vi "SwerveDriveTwoDrivers.vi"(0 "Strafe Joystick Axes":cluster{"X":dbl, "Y":dbl}, 1 "Face Joystick Axes":cluster{"X":dbl, "Y":dbl}, 2 "Trigger Axes":cluster{"output":dbl, dbl}, 3 "Face PID Gains":T2 {"derivative time (Td, min)" format="%.3f"; "integral time (Ti, min)" format="%.3f"; "proportional gain (Kc)" format="%.3f"}, 4 "Angle (degrees; 0 = right)":dbl, 5 "error in (no error)":errorcluster, 6 "Strafe Multiplier":dbl, 8 "Rotation Multiplier":dbl, 9 "ArmCRotates?":bool, 10 "Max Wheel Speed":dbl) -> (19 "error out":errorcluster)   [LabVIEW 2014]
uses:
  <vilib>/addons/control/pid/pid.llb/PID Control Input Filter (DBL).vi
  <vilib>/addons/control/pid/pid.llb/PID (DBL).vi
  <vilib>/addons/control/pid/NI_PID_pid.lvlib
panel:
  out "diff.":dbl
  out "Waveform Chart":T1(graph)
  out "Robot Heading":dbl(knob) scale=3.1416..-3.1416
  out "Joystick Angle":dbl(knob) scale=3.1416..-3.1416
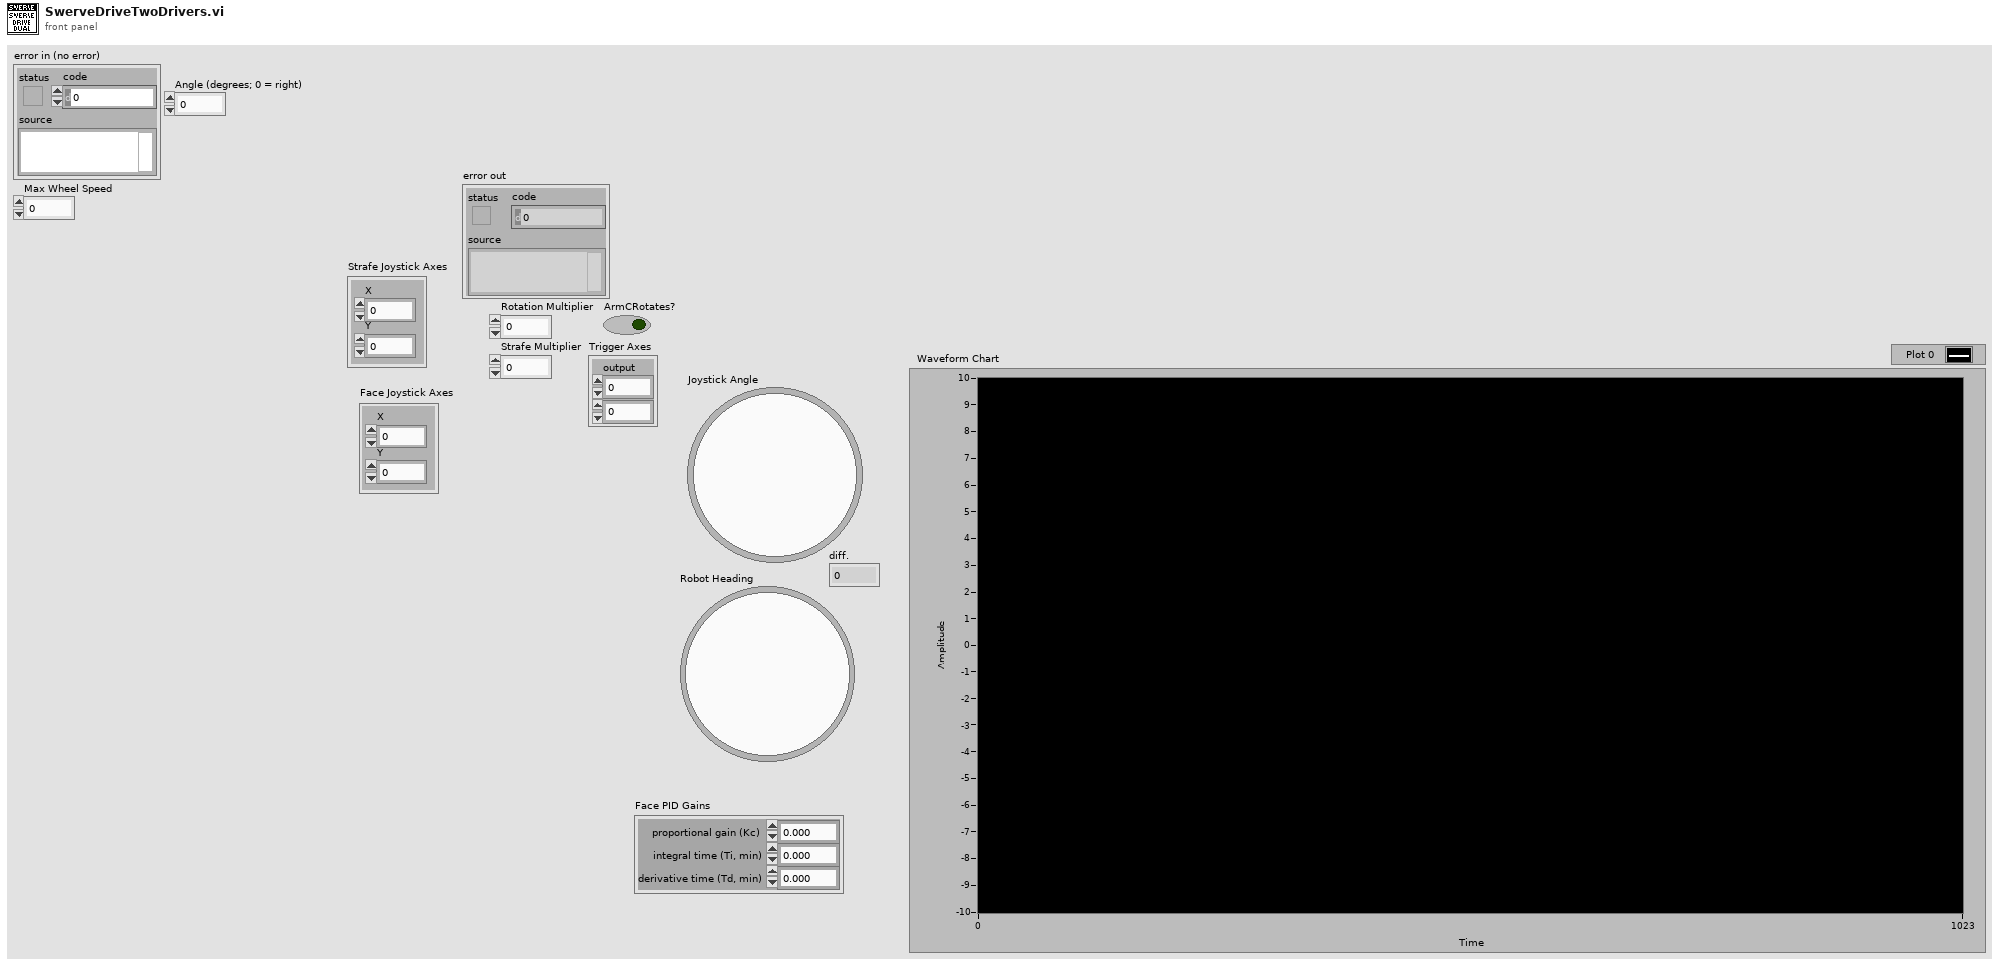
[diagram p1: front panel]
types:
  T1 = cluster{"output":dbl, "output":dbl, "millisecond timer value":u32}
  T2 = cluster{"proportional gain (Kc)":dbl, "integral time (Ti, min)":dbl, "derivative time (Td, min)":dbl}
  T3 = cluster{"output angle":dbl, "output":dbl, "millisecond timer value":u32}
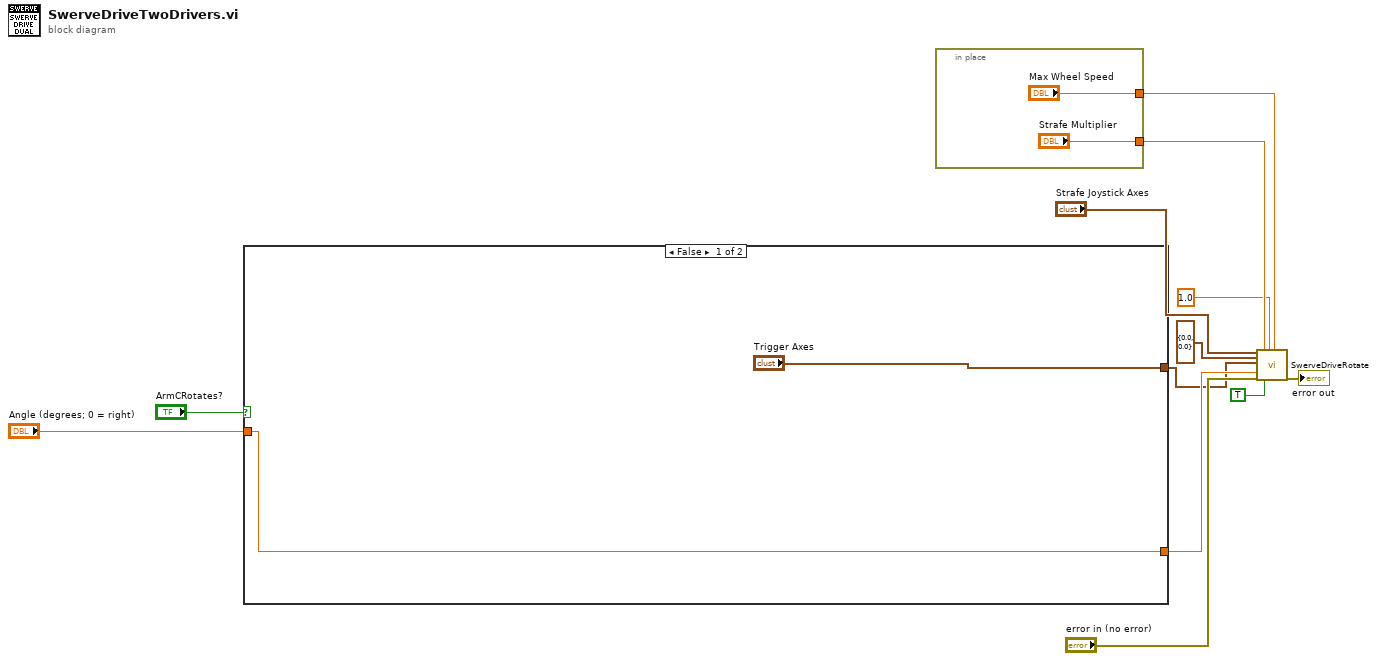
[diagram p0: block diagram]
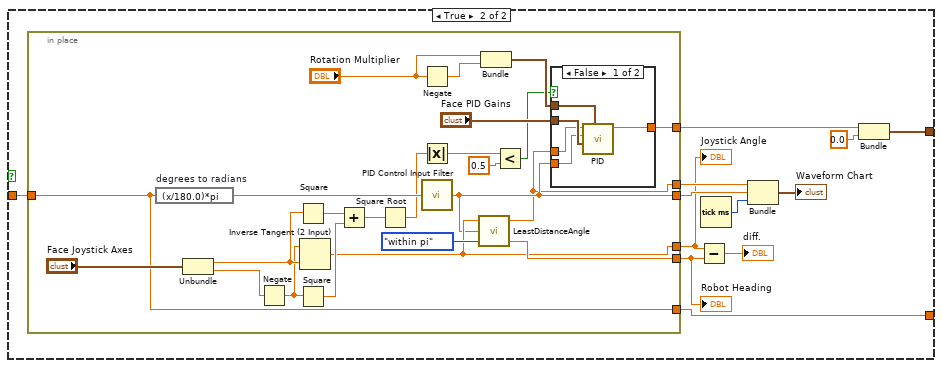
[diagram p2: hidden frame]
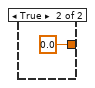
[diagram p3: hidden frame]
diagram:
  n1 = case shown="False" "ArmCRotates?" {
    tunnel: ["Trigger Axes" w24] -> w1
    tunnel: [w14 w23] -> w11
    tunnel: "Angle (degrees; 0 = right)" -> [w14 w15]
    frame False {
    }
    frame True {
      n2 = in-place {
        in-place-border: [w49] -> w25
        in-place-border: [w27] -> w23
        in-place-border: [w31] -> w18
        in-place-border: [w33] -> w17
        in-place-border: [w29] -> w20
        in-place-border: [w28] -> w19
        in-place-border: w15 -> [w27]
        n3 = expression code="(x/180.0)*pi" "degrees to radians"(w27) -> (w46:dbl)
        n4 = Unbundle("Face Joystick Axes") -> ("X"=w41:dbl, "Y"=w40:dbl)
        n5 = Negate(x=w40) -> (-x=w37:dbl)
        n6 = Square(x=w41) -> (x^2=w45:dbl)
        n7 = Square(x=w37) -> (x^2=w44:dbl)
        n8 = Inverse Tangent (2 Input)(1:w41, 2:w37) -> (0:w31:dbl)
        n9 = Add(x=w45, y=w44) -> (x+y=w43:dbl)
        n10 = Square Root(x=w43) -> (sqrt(x)=w42:dbl)
        n11 = Negate(x="Rotation Multiplier") -> (-x=w35:dbl)
        n12 = Absolute Value(x=w42) -> (abs(x)=w38:dbl)
        n13 = call-poly <vilib>:"PID Control Input Filter.vi"("input"=w46) -> ("output"=w29:dbl)  [unwired: 4 in]
        n14 = call "LeastDistanceAngle.vi"("Enum"=enum16{"within pi", "within pi/2"}."within pi", "Current angle"=w29, "target angle (between pi and -pi) 2"=w31) -> ("current angle (between pi and -pi) 2"=w33:dbl, "output angle"=w28:dbl)  [unwired: 1 out]
        n15 = Bundle("Rotation Multiplier"="Rotation Multiplier", w35) -> (w34:cluster{"Rotation Multiplier":dbl, dbl})  [unwired: 1 in]
        n16 = Less?(x=w38, y=0.5) -> (x < y?=w30:bool)
        n17 = case shown="False" w30 {
          tunnel: [w54 0.0 ("output")] -> w49
          tunnel: "Face PID Gains" -> [w53 _]
          tunnel: w34 -> [w52 _]
          tunnel: w29 -> [w51 _]
          tunnel: w28 -> [w50 _]
          frame False {
            n18 = call-poly <vilib>:"PID.vi"("output range"=w52, "PID gains"=w53, "process variable"=w51, "setpoint"=w50) -> ("output"=w54:dbl)  [unwired: 6 in, 1 out]
          }
          frame True {
          }
        }
      }
      "Joystick Angle" <- w18
      "Robot Heading" <- w17
      n19 = Subtract(x=w18, y=w17) -> (x-y=→"diff.":dbl)
      n20 = Tick Count (ms)() -> (millisecond timer value=w22:u32)
      n21 = Bundle("output angle"=w19, "output"=w20, "millisecond timer value"=w22) -> (→"Waveform Chart":T3)  [unwired: 1 in]
      n22 = Bundle("output"=w25, 0.0) -> (w24:cluster{"output":dbl, dbl})  [unwired: 1 in]
    }
  }
  n23 = in-place {
    in-place-border: ["Max Wheel Speed"] -> w7
    in-place-border: ["Strafe Multiplier"] -> w6
  }
  n24 = call "SwerveDriveRotate.vi"("Strafe Joystick Axes"="Strafe Joystick Axes", "Center of Rotation Joystick Axes"=cluster{"X":dbl, "Y":dbl} {"X"=0.0, "Y"=0.0}, "Trigger Axes"=w1, "Angle (degrees; 0 = right)"=w11, "error in (no error)"="error in (no error)", "Strafe Multiplier"=w6, "FieldCentric? (T)"=TRUE, "Rotation Multiplier"=1.0, "Max Wheel Speed"=w7) -> ("error out"=→"error out":errorcluster)  [unwired: 10 in]
